vi "findleftmostbitI16w.vi"(11 "number":i16 format="%b") -> (3 "Numeric":i16)   [LabVIEW 2018, in "posit.lvlib"]
uses:
  posit.lvlib
  <vilib>/rvi/Emulation/niFpgaGetClockAttributes.vi
  <vilib>/rvi/Emulation/niFpgaSctlEmulationGetInTimedLoop.vi
  <vilib>/rvi/Emulation/niFpgaEmulationReportErrorSimple.vi
  <vilib>/rvi/Emulation/niFpgaCriticalErrorInLSC.vi
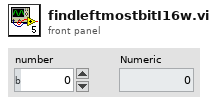
[diagram p1: front panel]
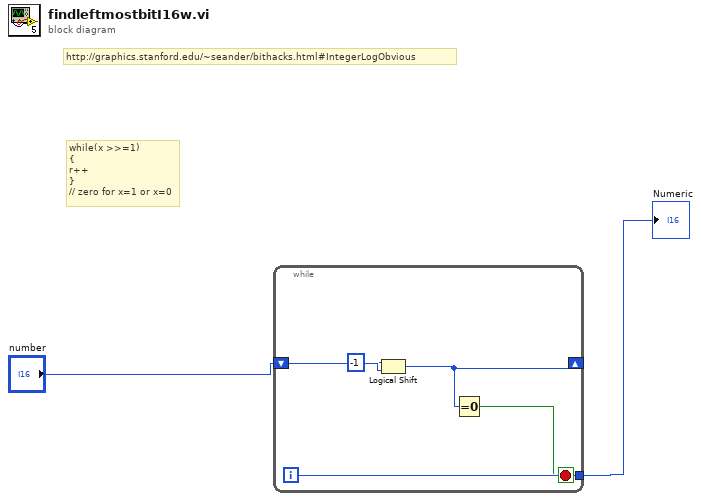
[diagram p0: block diagram]
diagram:
  # "while(x >>=1)\n{\nr++\n}\n// zero for x=1 or x=0"
  # "http://graphics.stanford.edu/~seander/bithacks.html#IntegerLogObvious"
  n1 = while {
    tunnel: [w7] -> w1
    shift-right: [w3] -> _
    shift-left: "number" -> [w6]
    i -> [w7]
    stop <- w4 stop-if-true
    n2 = Logical Shift(y=i16 -1, x=w6) -> (x << y=w3:i16)
    n3 = Equal To 0?(x=w3) -> (x = 0?=w4:bool)
  }
  "Numeric" <- w1
